vi "resetView.vi"(8 "error in (no error)":errorcluster, 11 "CategoryListUIAdapter in":refnum<class "CategoryListUIAdapter.lvclass">) -> (0 "error out":errorcluster, 3 "CategoryListUIAdapter out":refnum<class "CategoryListUIAdapter.lvclass">)   [LabVIEW 2018, in "CategoryListUIAdapter.lvclass"]
uses:
  CategoryListUIAdapter.lvclass
  <vilib>/Utility/miscctls.llb/LVRowAndColumnUnsignedTypeDef.ctl
  CategoryListUIAdapter.lvclass/CategoryListUIAdapter.ctl
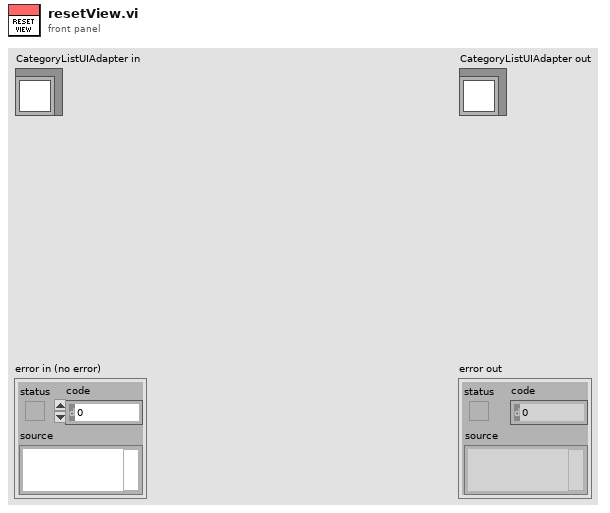
[diagram p1: front panel]
types:
  T1 = typedef "LVRowAndColumnUnsignedTypeDef.ctl" = cluster{"Row":u32, "Column":u32}
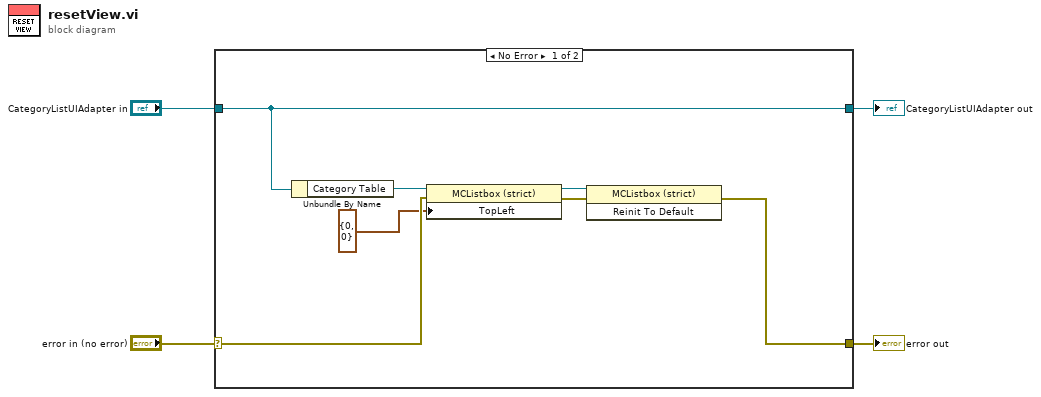
[diagram p0: block diagram]
diagram:
  n1 = case shown="No Error" "error in (no error)" {
    selector: "error in (no error)" -> [w7 w13]
    tunnel: [w6 w13] -> w3
    tunnel: [w11 w12] -> w1
    tunnel: "CategoryListUIAdapter in" -> [w11 w12]
    frame No Error {
      n2 = Unbundle By Name(w11) -> ("Category Table"=w10:refnum<vi>)
      n3 = property class="MCListbox (strict)"(reference=w10, error in=w7, "TopLeft"=T1 {"Row"=0, "Column"=0} ("Top Left Visible Cell")) -> (reference out=w9:refnum<vi>, error out=w8:errorcluster)
      n4 = invoke class="MCListbox (strict)" method="Reinit To Default"(reference=w9, error in=w8) -> (error out=w6:errorcluster)  [unwired: 1 in, 2 out]
    }
    frame Error {
    }
  }
  "error out" <- w3
  "CategoryListUIAdapter out" <- w1
